vi "Dashboard Main.vi"() -> ()   [LabVIEW 2015]
uses:
  <vilib>/Utility/miscctls.llb/LVRowAndColumnTypeDef.ctl
  <vilib>/event_ctls.llb/eventvkey.ctl
  <vilib>/Rock Robotics/WPI/Dashboard/WPI_DashboardLogging Global.vi
  <vilib>/Rock Robotics/Network Tables/NT Read Numeric Array.vi
  <vilib>/Rock Robotics/Network Tables/NT Read Boolean.vi
  <vilib>/Utility/config.llb/Write Key (String).vi
  <vilib>/Utility/config.llb/Write Key (I32).vi
  <vilib>/Utility/config.llb/NI_LVConfig.lvlib
panel:
  in  "TCP":refnum<k5>
  in  "Rec Mode":enum32{"Stop", "Record", "Playback"}(radio)
  in  "Vision":u16(ring) items=["Camera Off", "USB Camera SW", "USB Camera HW", "IP Camera"]
  out "Camera IP":string
  out "Image Message":string="Timeout in Camera Communications"
  in  "Dashboard Tab":T1(tab)
  in  "Select Auto":string(combo)
  out "NT Connection":bool
  in  "Camera Settings":T2={"Frame Rate"=30, "Compression"=30, "Size"=1} {"Frame Rate" scale=1.0..30.0; "Size" items=["640x480", "320x240", "160x120"]}
  out "MotorChart R":cluster{"Numeric":dbl, "Numeric":dbl}(graph)
  out "MotorChart L":T3(graph)
  out "MotorSliders R":cluster{"MotorSlide1":dbl, "MotorSlide2":dbl} {"MotorSlide2" scale=-1.0..1.0 scale format="%#_2e"; "MotorSlide1" scale=-1.0..1.0 scale format="%#_2e"}
  out "MotorSliders L":T4 {"MotorSlide4 2" scale=0.0..14.0 scale format="%#_2e"; "MotorSlide2" scale=-1.0..1.0 scale format="%#_2e"; "MotorSlide1" scale=-1.0..1.0 scale format="%#_2e"}
  out "Gyro":dbl(knob) scale=0.0..360.0
  out "JS1 Z":dbl(slide) scale=-1.0..1.0 scale format="%#_2e"
  out "JS1 Graph":cluster{"X":dbl, "Y":dbl}[](graph)
  out "JS1 Buttons":T5
  out "JS2 Z":dbl(slide) scale=-1.0..1.0 scale format="%#_2e"
  out "JS2 Graph":cluster{"X":dbl, "Y":dbl}[](graph)
  out "JS2 Buttons":T5
  out "Mode":T6(ring)=enum."Auto Disabled"
  in  "DB Camera Config":bool
  out "fps":dbl format="%#.1g"
  out "Mbps":dbl format="%#.1g"
  out "Mbps LED":bool
  in  "DB/String 9":string
  in  "DB/String 8":string
  in  "DB/String 7":string
  in  "DB/String 6":string
  in  "DB/String 5":string
  in  "DB/String 4":string
  in  "DB/String 3":string
  in  "DB/String 2":string
  in  "DB/String 1":string
  in  "DB/String 0":string
  in  "DB/Slider 0":dbl(slide) scale=0.0..5.0
  in  "DB/Slider 1":dbl(slide) scale=0.0..5.0
  in  "DB/Slider 2":dbl(slide) scale=0.0..5.0
  in  "DB/Slider 3":dbl(slide) scale=0.0..5.0
  out "DB/LED 3":bool
  out "DB/LED 2":bool
  out "DB/LED 1":bool
  out "DB/LED 0":bool
  in  "DB/Button 3":bool
  in  "DB/Button 2":bool
  in  "DB/Button 1":bool
  in  "DB/Button 0":bool caption="New Name"
  out "Target In Range":bool
  out "Target Found":bool
  out "Auto Aim Running":bool
  out "Target Position":string
  out "Target Distance":dbl
  in  "Auto Select":i32(knob) scale=0.0..10.0
  out "Shooter Ready":bool
  out "Vision FPS":dbl
  out "Auto Aim Ready":bool
  in  "Test Slider":dbl(slide) scale=0.0..100.0 scale format="%#_3g"
  in  "On/Off":bool caption="Solenoid"
  in  "Test Name":u16(ring) items=["Select the test to run..."]
  in  "Test Tree":string(tree)
  in  "Motor":cluster{"Value":dbl, "Enable":bool} {"Value" scale=-1.0..1.0 scale format="%#_3g"}
  out "Progress":T7 {"Test Progress" scale=0.0..100.0}
  in  "Rev/Fwd":cluster{"Forward":bool, "Reverse":bool}
  in  "Test Ring":u16(ring) items=["Monochrome", "Color"]
  out "Cmd Status":string
  in  "Execute Command":bool
  in  "Command Params":string[][](table)
  in  "Command Selection":i32(listbox)
  in  "CheckList":i32(listbox)
  out "Tree":string(tree)
  out "Camera Image":T8(plugin-control)
  out "Background":bool
  # "Left"
  # "Front"
  # "Right"
  # "Battery"
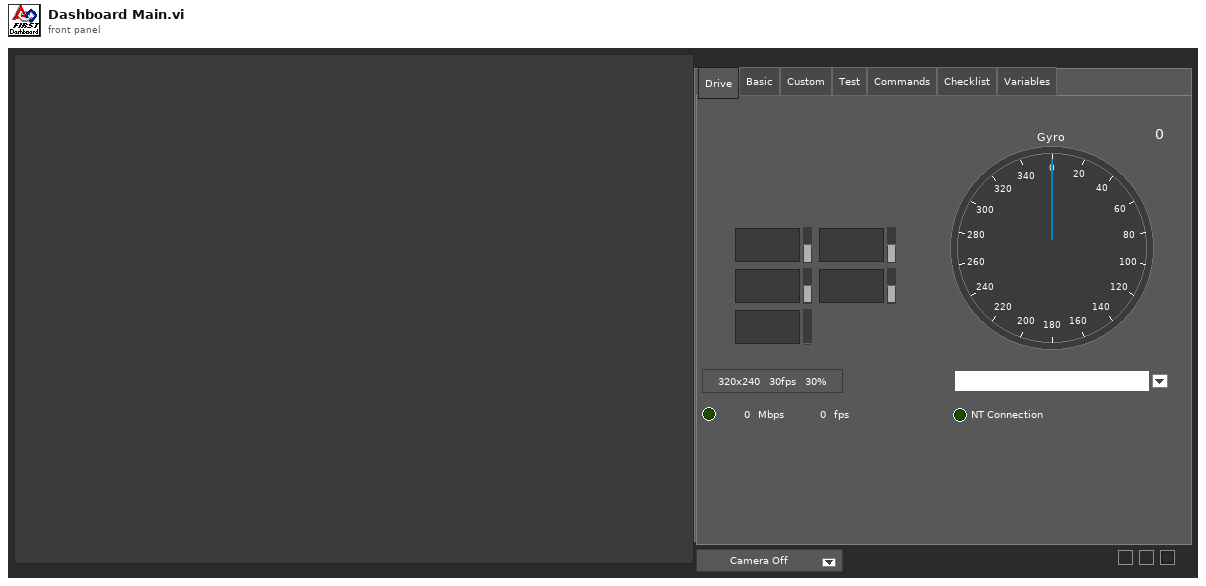
[diagram p1: front panel]
types:
  T1 = enum32{"Drive", "Basic", "Custom", "Test", "Commands", "Checklist", "Variables"}
  T2 = cluster{"Frame Rate":i32, "Compression":i32, "Size":u16}
  T3 = cluster{"Numeric":dbl, "Numeric":dbl, "Battery V":dbl}
  T4 = cluster{"MotorSlide1":dbl, "MotorSlide2":dbl, "MotorSlide4 2":dbl}
  T5 = cluster{bool, bool, bool, bool, bool, bool, bool, bool, bool, bool, bool, bool}
  T6 = enum8{"Tele-Op Disabled", "Tele-Op Enabled", "Auto Disabled", "Auto Enabled", "Test Disabled", "Test Enabled", "Disconnected", "No Code", "E-Stop"}
  T7 = cluster{"Test Progress":u8, "Test Progress Text":string}
  T8 = typedef "IMAQ Image.ctl" = refnum<image>
  T9 = cluster{"IDs":cluster{"RPC field ID":u16, "Unique ID":u16}, "String":string}
  T10 = enum32{"Drive", "Basic", "Custom", "Test", "Checklist", "Variables"}
  T11 = typedef "Image Type" = u32
  T12 = cluster{"Camera Image":refnum<vi>, "Dashboard Tab":refnum<vi>, "Background":refnum<vi>, "Vision":refnum<vi>, "Rec Mode":refnum<vi>, "Test Slider":refnum<vi>, "On/Off ":refnum<vi>, "Test Ring":refnum<vi>, "Rev/Fwd":refnum<vi>, "Test Name":refnum<vi>, "Motor":refnum<vi>, "Progress":refnum<vi>, "CheckList":refnum<vi>, "Tree":refnum<vi>, "Test Tree":refnum<vi>, "Command Params":refnum<vi>, "Command Selection":refnum<vi>, "Execute Command":refnum<vi>, "Cmd Status":refnum<vi>}
  T13 = cluster{"Error Strings":string, "Disable Counts":cluster{u16, u16}, "Rail Faults":cluster{u16, u16, u16}, "Robot IP":string, "DB Mode":u8, "Event Info":cluster{"Name":string, "Type":u8, "Number":u16, "Replay":u8}, "Camera Addr":string}
  T14 = cluster{"Storage":cluster{"Disk Free":u64, "RAM Block":u32, "RAM free":u32}, "CPU Utilization":cluster{"CPU % ISR":sgl, "CPU % Time Crit":sgl, "CPU % Timed Str":sgl, "CPU % High":sgl, "CPU % Above":sgl, "CPU % Normal":sgl, "CPU % Low":sgl}, "CAN":cluster{"% Bus Utilization":sgl, "Bus Off Cnt":u32, "TX_FIFO Full Cnt":u32, "Receive Error Cnt":u8, "Transmit Error Cnt":u8}, "HID":cluster{"HID Outputs":u32, "Rumble Low":u16, "Rumble High":u16}[]}
  T15 = cluster{"Status bits":cluster{"Test Mode":bool, "Autonomous":bool, "Enabled":bool, "Code Start":bool, "Brownout":bool, "Reserved 2":bool, "Reserved 3":bool, "E-Stop":bool}, "Code Trace":cluster{"Disabled":bool, "TeleOp":bool, "Auto":bool, "Test":bool}, "Controller Type":enum16{"unknown", "cRIO", "roboRio"}, "Code?":enum16{"unknown", "noCode", "code"}, "Battery V":dbl}
  T16 = cluster{"Control Bits":cluster{"TestMode":bool, "Autonomous":bool, "Enabled":bool, "FMS Present":bool, bool, bool, bool, "E-Stop":bool}, "Team Station ":u8, "Countdown":sgl, "Joystick Values":cluster{"Axes":dbl[], "Buttons":bool[], "POVs":i16[]}[]}
  T17 = cluster{"Axes":dbl[], "Buttons":bool[], "POVs":i16[]}[]
  T18 = cluster{"Axes":dbl[], "Buttons":bool[], "POVs":i16[]}
  T19 = cluster{"Buttons[0]":bool, "Buttons[1]":bool, "Buttons[2]":bool, "Buttons[3]":bool, "Buttons[4]":bool, "Buttons[5]":bool, "Buttons[6]":bool, "Buttons[7]":bool, "Buttons[8]":bool, "Buttons[9]":bool, "Buttons[10]":bool, "Buttons[11]":bool}
  T20 = typedef "NI_LVConfig.lvlib/Config Data RefNum.ctl" = refnum<k1>
  T21 = cluster{"Operation":enum16{"Update", "Clear"}, "Color Box":u32}[]
  T22 = typedef "eventvkey.ctl" = enum16{"ASCII", "Enter", "Return", "Shift", "Ctrl", "Alt", "Cmd", "Opt", "Caps", "NumLock", "Clear", "Break", "Up", "Down", "Left", "Right", "Insert", "Delete", "Home", "End", "PageUp", "PageDown", "Escape", "Help", "Pause", "ScrollLock", "F1", "F2", "F3", "F4", "F5", "F6", "F7", "F8", "F9", "F10", "F11", "F12", "F13", "F14", "F15", "F16", "F17", "F18", "F19", "F20", "F21", "F22", "F23", "F24", "Play", "VolumeUp", "VolumeDown", "Mute", "Two Byte Char"}
  T23 = cluster{"Image Size":bool, "Image Type":bool, "Pixel Value":bool, "ROI Information":bool, "Zoom Factor":bool}
  T24 = enum8{"Enabled", "Disabled", "Disabled and Grayed Out"}
  T25 = cluster{"Operation":enum16{"Update", "Clear"}, "Color Box":u32}
  T26 = typedef "LVRowAndColumnTypeDef.ctl" = cluster{"Row":i32, "Column":i32}
  T27 = cluster{"Shift":bool, "Ctrl":bool, "Alt":bool, "Cmd":bool, "Opt":bool}
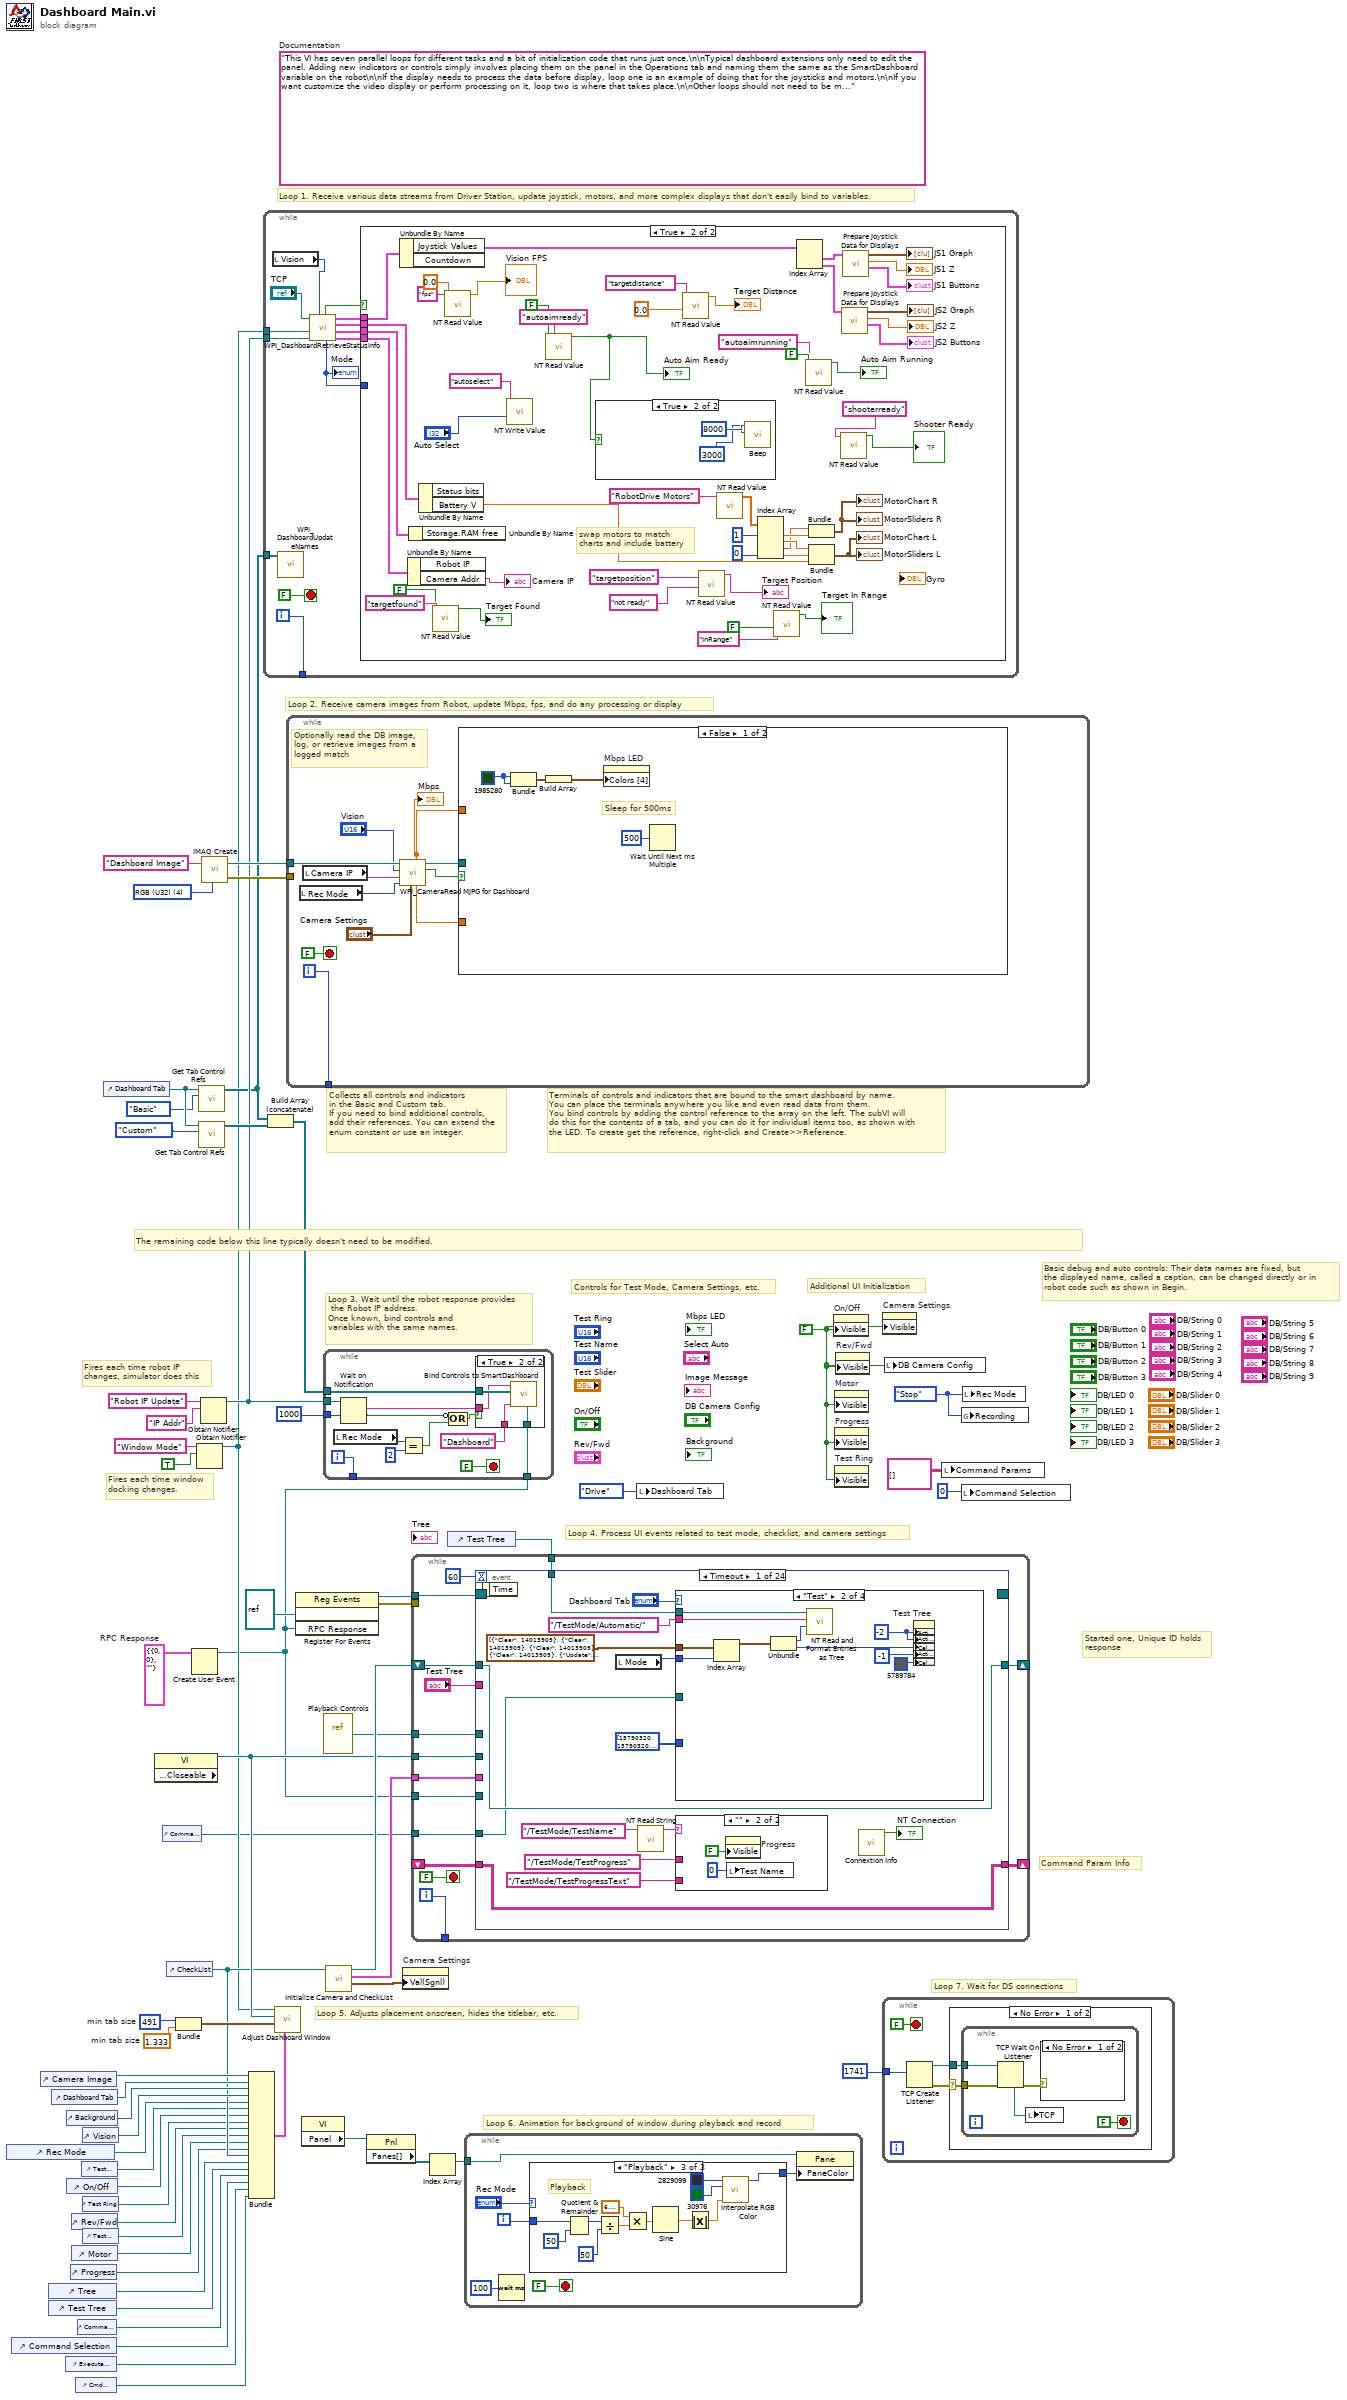
[diagram p0: block diagram]
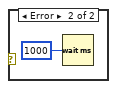
[diagram p2: hidden frame]
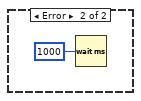
[diagram p3: hidden frame]
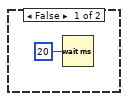
[diagram p4: hidden frame]
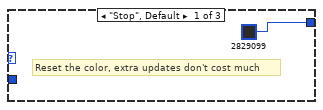
[diagram p6: hidden frame]
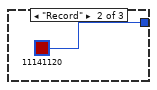
[diagram p7: hidden frame]
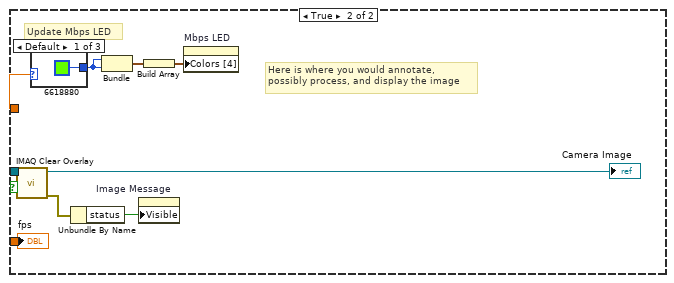
[diagram p9: hidden frame]
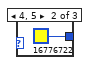
[diagram p10: hidden frame]
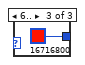
[diagram p11: hidden frame]
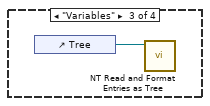
[diagram p13: hidden frame]
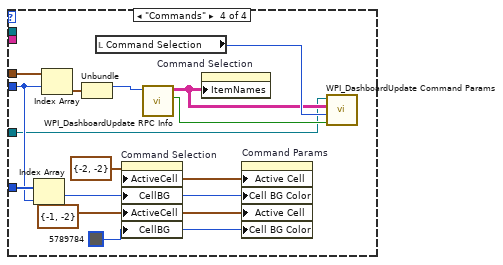
[diagram p14: hidden frame]
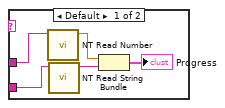
[diagram p15: hidden frame]
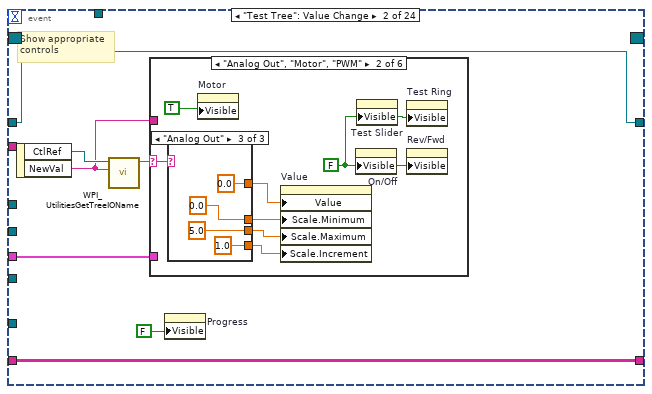
[diagram p16: hidden frame]
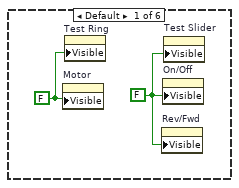
[diagram p17: hidden frame]
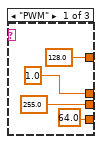
[diagram p18: hidden frame]
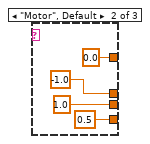
[diagram p19: hidden frame]
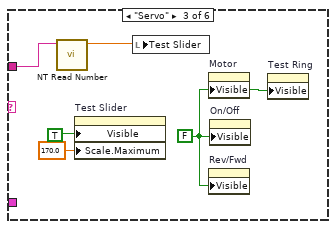
[diagram p20: hidden frame]
diagram:
  w7 = T9 {"IDs"={"RPC field ID"=0, "Unique ID"=0}, "String"=""}  # RPC Response
  w33 = 491  # min tab size
  w32 = 1.333  # min tab size
  w41 = enum32{"Stop", "Record", "Playback"}."Stop" ("Rec Mode")
  w15 = FALSE ("Visible")
  (unwired) "This VI has seven parallel loops for different tasks and a bit of initialization code that runs just once.\n\nTypical dashboard extensions only need to edit the panel. Adding new indicators or controls simply involves placing them on the panel in the Operations tab and naming them the same as the SmartDashboard variable on the robot\n\nIf the display needs to process the data before display, loop one is an example of doing that for the joysticks and motors.\n\nIf you want customize the video display or perform processing on it, loop two is where that takes place.\n\nOther loops should not need to be modified. They are pretty standard, and document the task they perform."  # Documentation
  w61 = T11 4 items=["Grayscale (U8)", "Grayscale (I16)", "Grayscale (SGL)", "Complex (CSG)", "RGB (U32)", "HSL (U32)", "RGB (U64)"] ("Image Type")
  # "Command Param Info"
  # "Started one, Unique ID holds\nresponse"
  # "Loop 7. Wait for DS connections"
  # "Basic debug and auto controls: Their data names are fixed, but\nthe displayed name, called a caption, can be changed directly or in\nrobot code such as shown in Begin."
  # "Controls for Test Mode, Camera Settings, etc."
  # "Additional UI Initialization"
  # "Loop 6. Animation for background of window during playback and record"
  # "Fires each time robot IP\nchanges, simulator does this"
  # "Fires each time window\ndocking changes."
  # "Collects all controls and indicators\nin the Basic and Custom tab.\nIf you need to bind additional controls,\nadd their references. You can extend the\nenum constant or use an integer."
  # "The remaining code below this line typically doesn't need to be modified."
  # "Loop 4. Process UI events related to test mode, checklist, and camera settings"
  # "Terminals of controls and indicators that are bound to the smart dashboard by name.\nYou can place the terminals anywhere you like and even read data from them.\nYou bind controls by adding the control reference to the array on the left. The subVI will\ndo this for the contents of a tab, and you can do it for individual items too, as shown with\nthe LED. To create get the reference, right-click and Create>>Reference."
  # "Loop 3. Wait until the robot response provides\n the Robot IP address.\nOnce known, bind controls and\nvariables with the same names."
  # "Loop 5. Adjusts placement onscreen, hides the titlebar, etc."
  # "Loop 1. Receive various data streams from Driver Station, update joystick, motors, and more complex displays that don't easily bind to variables."
  # "Loop 2. Receive camera images from Robot, update Mbps, fps, and do any processing or display"
  n1 = control-ref of="Rec Mode"() -> (w21:refnum<vi>)
  n2 = control-ref of="Command Selection"() -> (w6:refnum<vi>)
  n3 = control-ref of="Camera Image"() -> (w36:refnum<vi>)
  n4 = control-ref of="Tree"() -> (w25:refnum<vi>)
  n5 = control-ref of="Test Tree"() -> (w24:refnum<vi>)
  n6 = control-ref of="Dashboard Tab"() -> (w35:refnum<vi>)
  n7 = control-ref of="Execute Command"() -> (w8:refnum<vi>)
  n8 = control-ref of="Background"() -> (w30:refnum<vi>)
  n9 = control-ref of="On/Off"() -> (w19:refnum<vi>)
  n10 = control-ref of="Progress"() -> (w16:refnum<vi>)
  n11 = control-ref of="Rev/Fwd"() -> (w17:refnum<vi>)
  n12 = control-ref of="Motor"() -> (w22:refnum<vi>)
  n13 = control-ref of="Cmd Status"() -> (w2:refnum<vi>)
  n14 = control-ref of="Command Params"() -> (w9:refnum<vi>)
  n15 = control-ref of="Test Slider"() -> (w20:refnum<vi>)
  n16 = control-ref of="Vision"() -> (w34:refnum<vi>)
  n17 = control-ref of="Test Ring"() -> (w18:refnum<vi>)
  n18 = control-ref of="Test Name"() -> (w23:refnum<vi>)
  n19 = control-ref of="Dashboard Tab"() -> (w39:refnum<vi>)
  n20 = property class="VI" props=["Front Panel.Closeable"]() -> (reference out=w40:refnum<vi>)  [unwired: 2 in, 2 out]
  n21 = control-ref of="Command Params"() -> (w1:refnum<vi>)
  n22 = control-ref of="CheckList"() -> (w26:refnum<vi>)
  n23 = Bundle("min tab size"=w33, "min tab size"=w32) -> (w31:cluster{"min tab size":i32, "min tab size":dbl})  [unwired: 1 in]
  n24 = Create User Event(user event datatype=w7) -> (user event=w3:refnum<user-event>)  [unwired: 1 in, 1 out]
  n25 = Obtain Notifier(name (unnamed)="Window Mode", notification data type=TRUE) -> (notifier out=w12:refnum<notifier>)  [unwired: 2 in, 2 out]
  n26 = call <vilib>:"Get Tab Control Refs.vi"("Page Index"=T10."Basic" ("Dashboard Tab"), "TabControl in"=w39) -> ("ControlsOnPage"=w13:refnum<vi>[])  [unwired: 9 in]
  n27 = call <vilib>:"Get Tab Control Refs.vi"("Page Index"=T10."Custom" ("Dashboard Tab"), "TabControl in"=w39) -> ("ControlsOnPage"=w38:refnum<vi>[])  [unwired: 9 in]
  n28 = Obtain Notifier(name (unnamed)="Robot IP Update", notification data type="IP Addr" ("name (unnamed)")) -> (notifier out=w14:refnum<notifier>)  [unwired: 2 in, 2 out]
  n29 = call "IMAQ Create"("Image Name"="Dashboard Image", "Image Type"=w61) -> ("New Image"=w59:T8, "error out"=w58:errorcluster)  [unwired: 2 in, 1 out]
  n30 = Bundle("Camera Image"=w36, "Dashboard Tab"=w35, "Background"=w30, "Vision"=w34, "Rec Mode"=w21, "Test Slider"=w20, "On/Off"=w19, "Test Ring"=w18, "Rev/Fwd"=w17, "Test Name"=w23, "Motor"=w22, "Progress"=w16, "CheckList"=w26, "Tree"=w25, "Test Tree"=w24, "Command Params"=w9, "Command Selection"=w6, "Execute Command"=w8, "Cmd Status"=w2) -> (w27:T12)  [unwired: 1 in]
  n31 = while {
    tunnel: [w73] -> _
    tunnel: w14 -> [w67]
    tunnel: w13 -> [w66]
    tunnel: w12 -> [w62]
    i -> [w73]
    stop <- FALSE stop-if-true
    n32 = local read "Vision"() -> (w64:u16)
    n33 = call <vilib>:"WPI_DashboardUpdateNames.vi"("Controls on Tab"=w66) -> ()  [unwired: 11 in]
    n34 = call <vilib>:"WPI_DashboardRetrieveStatusInfo.vi"("Vision"=w64, "Binding Refnum"=w67, "Window Mode Notifier"=w62, "TCP Cnx"="TCP") -> ("Power and Errors"=w68:T13, "Robot Metrics"=w71:T14, "Status Info"=w72:T15, "Control Info"=w69:T16, "Robot Mode"=w65:T6, "Process?"=w70:bool)  [unwired: 2 in]
    "Mode" <- w65
    n35 = case shown="True" w70 {
      tunnel: w72 -> [_ w125]
      tunnel: w71 -> [_ w124]
      tunnel: w69 -> [_ w123]
      tunnel: w68 -> [_ w122]
      tunnel: w65 -> [_ _]
      frame False {
        n36 = Wait (ms)(milliseconds to wait=u32 20) -> ()  [unwired: 1 out]
      }
      frame True {
        # "swap motors to match\ncharts and include battery"
        n37 = Unbundle By Name(w123) -> ("Joystick Values"=w112:T17)  [unwired: 1 out]
        n38 = Unbundle By Name(w122) -> ("Camera Addr"=→"Camera IP":string)  [unwired: 1 out]
        n39 = Unbundle By Name(w124) -> ()  [unwired: 1 out]
        n40 = Unbundle By Name(w125) -> ("Battery V"=w113:dbl)  [unwired: 1 out]
        n41 = call-poly <vilib>:"NT Read Value.vi"("Default Value"=FALSE, "Name"="targetfound") -> ("Boolean"=→"Target Found":bool)  [unwired: 8 in, 1 out]
        n42 = call-poly <vilib>:"NT Read Value.vi"("Default Value"=0.0, "Name"="fps") -> ("Numeric"=→"Vision FPS":dbl)  [unwired: 8 in, 1 out]
        n43 = call-poly <vilib>:"NT Write Value.vi"("Numeric"="Auto Select", "Name"="autoselect") -> ()  [unwired: 9 in, 1 out]
        n44 = call-poly <vilib>:"NT Read Value.vi"("Default Value"=FALSE, "Name"="autoaimready") -> ("Boolean"=w97:bool)  [unwired: 8 in, 1 out]
        "Auto Aim Ready" <- w97
        n45 = case shown="True" w97 {
          frame False {
          }
          frame True {
            n46 = call <vilib>:"Beep.vi"("duration (msec)"=3000, "frequency (Hz)"=8000) -> ()  [unwired: 10 in]
          }
        }
        n47 = call-poly <vilib>:"NT Read Value.vi"("Default Value"=0.0, "Name"="targetdistance") -> ("Numeric"=→"Target Distance":dbl)  [unwired: 8 in, 1 out]
        n48 = call-poly <vilib>:"NT Read Value.vi"("Default Value"="not ready", "Name"="targetposition") -> ("String"=→"Target Position":string)  [unwired: 8 in, 1 out]
        n49 = call-poly <vilib>:"NT Read Value.vi"("Name"="RobotDrive Motors") -> ("Numeric Array"=w101:dbl[])  [unwired: 9 in, 1 out]
        n50 = Index Array(array=w101, index #1=1, index #4=0) -> (element #1=w117:dbl, element #2=w118:dbl, element #3=w116:dbl, element #4=w121:dbl)  [unwired: 2 in]
        n51 = call-poly <vilib>:"NT Read Value.vi"("Default Value"=FALSE, "Name"="InRange") -> ("Boolean"=→"Target In Range":bool)  [unwired: 8 in, 1 out]
        n52 = Index Array(array=w112) -> (element #1=w111:T18, element #2=w106:T18)  [unwired: 2 in]
        n53 = call-poly <vilib>:"NT Read Value.vi"("Default Value"=FALSE, "Name"="autoaimrunning") -> ("Boolean"=→"Auto Aim Running":bool)  [unwired: 8 in, 1 out]
        n54 = Bundle("Numeric"=w116, "Numeric"=w117) -> (→"MotorChart R" →"MotorSliders R":cluster{"Numeric":dbl, "Numeric":dbl})  [unwired: 1 in]
        n55 = Bundle("Numeric"=w118, "Numeric"=w121, "Battery V"=w113) -> (→"MotorChart L" →"MotorSliders L":T3)  [unwired: 1 in]
        n56 = call-poly <vilib>:"NT Read Value.vi"("Name"="shooterready") -> ("Boolean"=→"Shooter Ready":bool)  [unwired: 9 in, 1 out]
        n57 = call "Prepare Joystick Data for Displays.vi"("Joystick Values"=w106) -> ("Buttons"=→"JS2 Buttons":T19, "Z Axis"=→"JS2 Z":dbl, "Cartesian Data"=→"JS2 Graph":cluster{"X axis":dbl, "X axis":dbl}[])  [unwired: 8 in]
        n58 = call "Prepare Joystick Data for Displays.vi"("Joystick Values"=w111) -> ("Buttons"=→"JS1 Buttons":T19, "Z Axis"=→"JS1 Z":dbl, "Cartesian Data"=→"JS1 Graph":cluster{"X axis":dbl, "X axis":dbl}[])  [unwired: 8 in]
      }
    }
  }
  n59 = Build Array (concatenate)(w13, w38) -> (w37:refnum<vi>[])
  n60 = call "Adjust Dashboard Window.vi"("Sizing Refnums"=w27, "Size Constraints"=w31, "VI"=w40, "WIn Mode"=w12) -> ()  [unwired: 8 in]
  n61 = while {
    tunnel: w59 -> [w136]
    tunnel: w58 -> [_]
    tunnel: [w137] -> _
    i -> [w137]
    stop <- FALSE stop-if-true
    # "Optionally read the DB image,\nlog, or retrieve images from a\nlogged match"
    n62 = local read "Rec Mode"() -> (w131:enum32{"Stop", "Record", "Playback"})
    n63 = local read "Camera IP"() -> (w129:string)
    n64 = call <vilib>:"WPI_CameraRead MJPG for Dashboard.vi"("Camera Settings"="Camera Settings", "Rec Mode"=w131, "Camera IP"=w129, "Camera Mode"="Vision", "Refnum in"=w136) -> ("Active"=w134:bool, "Refnum out"=w135:T8, "FPS"=w133:dbl, "Bandwidth (Mbps)"=w128:dbl)  [unwired: 3 in]
    "Mbps" <- w128
    n65 = case shown="False" w134 {
      tunnel: w135 -> [_ w146]
      tunnel: w128 -> [_ w145]
      tunnel: w133 -> [_ w143]
      frame False {
        w139 = u32 1985280 ("Color Box")
        # "Sleep for 500ms"
        n66 = Bundle("Color Box"=w139, "Color Box"=w139) -> (w141:cluster{"Color Box":u32, "Color Box":u32})  [unwired: 1 out]
        n67 = Build Array(w141) -> (w140:cluster{"Color Box":u32, "Color Box":u32}[])
        n68 = property on="Mbps LED" class="Bool (strict)"("Colors [4]"=w140) -> ()  [unwired: 2 in, 2 out]
        n69 = Wait Until Next ms Multiple(millisecond multiple=u32 500) -> ()  [unwired: 1 out]
      }
      frame True {
        # "Here is where you would annotate,\npossibly process, and display the image"
        # "Update Mbps LED"
        n70 = call "IMAQ Clear Overlay"("Image"=w146) -> ("error out"=w150:errorcluster, "Image Out"=→"Camera Image":T8)  [unwired: 2 in, 7 out]
        n71 = case shown="Default" w145 {
          tunnel: [u32 6618880 ("Color Box") u32 16776722 ("Color Box") u32 16716800 ("Color Box")] -> w147
          frame Default {
          }
          frame 4, 5 {
          }
          frame 6.. {
          }
        }
        n72 = Unbundle By Name(w150) -> ("status"=w151:bool)
        n73 = Bundle("Color Box"=w147, "Color Box"=w147) -> (w149:cluster{"Color Box":u32, "Color Box":u32})  [unwired: 1 out]
        n74 = property on="Image Message" class="Str"("Visible"=w151) -> ()  [unwired: 2 in, 2 out]
        n75 = Build Array(w149) -> (w148:cluster{"Color Box":u32, "Color Box":u32}[])
        n76 = property on="Mbps LED" class="Bool (strict)"("Colors [4]"=w148) -> ()  [unwired: 2 in, 2 out]
        "fps" <- w143
      }
    }
  }
  n77 = register-events(refnum<vi> refnum, w3) -> (reference out=w45:refnum<event-registration>, error out=w44:errorcluster)  [unwired: 2 in]
  n78 = property class="VI"() -> ("Panel"=w48:refnum<vi>)  [unwired: 2 in, 2 out]
  n79 = while {
    tunnel: w37 -> [w167]
    tunnel: w14 -> [w165]
    tunnel: [w163] -> _
    tunnel: u32 1000 ("milliseconds to wait") -> [w162]
    tunnel: w3 -> [w155]
    i -> [w163]
    stop <- FALSE stop-if-true
    n80 = local read "Rec Mode"() -> (w158:enum32{"Stop", "Record", "Playback"})
    n81 = Wait on Notification(notifier=w165, timeout in ms (-1)=w162) -> (notification=w164:string, timed out?=w160:bool)  [unwired: 2 in, 2 out]
    n82 = Equal?(x=w158, y=u16 2 ("Rec Mode")) -> (x = y?=w159:bool)
    n83 = Compound Arithmetic op=OR(invert w160, w159) -> (w161:bool)
    n84 = case shown="True" w161 {
      tunnel: w167 -> [_ w171]
      tunnel: w164 -> [_ w170]
      tunnel: "Dashboard" -> [_ w169]
      tunnel: w155 -> [_ w168]
      frame False {
      }
      frame True {
        n85 = call <vilib>:"Bind Controls to SmartDashboard.vi"("RPC ref"=w168, "Client Name"=w169, "Bound Control Refs"=w171, "Server IP Address"=w170) -> ()  [unwired: 8 in]
      }
    }
  }
  n86 = vi-ref "Playback Controls.vi"() -> (w46:refnum<vi>)
  n87 = call "Initialize Camera and CheckList.vi"("ListBox in"=w26) -> ("Cluster"=w52:cluster{"value":i32, "value":i32, "index":i32}, "Array"=w53:cluster{string[]}[], "File Refnum"=w51:T20)  [unwired: 8 in]
  n88 = property class="Pnl"(reference=w48) -> ("Panes[]"=w49:refnum<vi>[])  [unwired: 1 in, 2 out]
  n89 = property on="Camera Settings" class="Clust (strict)"("Val(Sgnl)"=w52) -> ()  [unwired: 2 in, 2 out]
  n90 = Index Array(array=w49) -> (element=w47:refnum<vi>)  [unwired: 1 in]
  n91 = control-ref of="Test Tree"() -> (w50:refnum<vi>)
  n92 = while {
    tunnel: w53 -> [w183]
    shift-right: [w182] -> _
    shift-left: w51 -> [w181]
    tunnel: [w180] -> _
    tunnel: w50 -> [w179]
    tunnel: w46 -> [w178]
    tunnel: w45 -> [w177]
    tunnel: w44 -> [_]
    tunnel: w40 -> [w176]
    tunnel: w3 -> [w175]
    tunnel: w1 -> [w174]
    shift-right: [w173] -> _
    shift-left: _ -> [w172]
    i -> [w180]
    stop <- FALSE stop-if-true
    n93 = event shown="[0] Timeout" {
      selector: w177 -> [_ _ _ _ _ _ _ _ _ _ _ _ _ _ _ _ _ _ _ _ _ _ _ _]
      dyn-events: [_ _ _ _ _ _ _ _ _ _ _ _ _ _ _ _ _ _ w492 _ _ _ _ _] -> _
      timeout: u32 60 ("milliseconds to wait") -> [_ _ _ _ _ _ _ _ _ _ _ _ _ _ _ _ _ _ _ _ _ _ _ _]
      tunnel: w179 -> [w196 _ _ _ _ _ _ _ _ _ _ _ _ _ _ _ _ _ _ _ _ _ _ _]
      tunnel: "Test Tree" -> [_ _ _ _ _ _ _ _ _ _ _ _ _ w455 w464 w467 w472 w481 _ _ _ _ _ _]
      tunnel: w183 -> [_ w234 _ _ _ _ _ _ _ _ _ w417 w448 _ _ _ _ _ _ _ _ _ _ _]
      tunnel: [w193 w233 w337 w343 w353 w357 w363 w375 w383 w389 w402 w416 w441 w454 w462 w466 w471 w480 w494 w510 w512 w520 w531 w536] -> w182
      tunnel: w181 -> [w193 w233 w337 w343 w353 w357 w363 w375 w383 w389 w402 w415 w441 w454 w462 w466 w471 w480 w494 w510 w512 w520 w531 w536]
      tunnel: w178 -> [_ _ _ _ _ _ _ _ _ _ _ _ _ _ _ _ _ _ w495 _ w515 _ _ _]
      tunnel: w176 -> [_ _ _ _ _ _ _ _ _ _ _ _ _ _ _ _ _ _ w490 _ _ _ _ _]
      tunnel: w175 -> [_ _ _ _ _ _ _ _ _ _ _ _ _ _ _ _ _ _ w486 _ _ _ _ _]
      tunnel: w174 -> [w188 _ _ _ _ _ w361 _ _ _ _ _ _ _ _ _ _ _ _ _ _ _ _ _]
      tunnel: [w187 w232 w336 w342 w352 w358 w359 w369 w380 w388 w401 w414 w440 w453 w461 w465 w470 w479 w485 w508 w511 w516 w524 w537] -> w173
      tunnel: w172 -> [w187 w232 w336 w342 w352 w358 w359 _ _ w388 w401 w414 w440 w453 w461 w465 w470 w479 w485 w508 w511 w516 w524 w537]
      event Timeout {
        n94 = event-data() -> ()  [unwired: 1 in, 1 out]
        n95 = local read "Mode"() -> (w190:T6)
        n96 = call <vilib>:"NT Read String.vi"("Name"="/TestMode/TestName") -> ("String"=w199:string)  [unwired: 9 in, 1 out]
        n97 = case shown="\"Test\"" "Dashboard Tab" {
          tunnel: w196 -> [_ w210 _ _]
          tunnel: "/TestMode/Automatic/" ("Name Pattern") -> [_ w209 _ _]
          tunnel: T21 [{"Operation"=enum."Clear", "Color Box"=14013909}, {"Operation"=enum."Clear", "Color Box"=14013909}, {"Operation"=enum."Clear", "Color Box"=14013909}, {"Operation"=enum."Clear", "Color Box"=14013909}, {"Operation"=enum."Update", "Color Box"=14013909}, {"Operation"=enum."Update", "Color Box"=16777215}, {"Operation"=enum."Clear", "Color Box"=14013909}, {"Operation"=enum."Clear", "Color Box"=14013909}, {"Operation"=enum."Clear", "Color Box"=14013909}] -> [_ w202 _ w219]
          tunnel: w190 -> [_ w201 _ w218]
          tunnel: u32[] [15790320, 15790320, 15790320, 15790320, 16777215, 16777215, 15790320, 15790320, 15790320] -> [_ _ _ w224]
          tunnel: w188 -> [_ _ _ w212]
          frame "Custom", Default {
          }
          frame "Test" {
            w208 = -2 ("Active Item:Row Number")
            n98 = Index Array(array=w202, index=w201) -> (element=w203:T25)
            n99 = Unbundle(w203) -> ("Operation"=w204:enum16{"Update", "Clear"}, "Color Box"=w205:u32)
            n100 = call <vilib>:"NT Read and Format Entries as Tree.vi"("Operation"=w204, "Name Pattern"=w209, "Tree Refnum"=w210) -> ()  [unwired: 7 in, 2 out]
            n101 = property on="Test Tree" class="Tree (strict)"("Active Item Row Number"=w208, "ActiveColNum"=w208, "CellBG"=w205, "Active Item Row Number"=-1 ("Active Item:Row Number"), "CellBG"=u32 5789784 ("Color Box")) -> ()  [unwired: 2 in, 2 out]
          }
          frame "Variables" {
            n102 = control-ref of="Tree"() -> (w211:refnum<vi>)
            n103 = call <vilib>:"NT Read and Format Entries as Tree.vi"("Tree Refnum"=w211) -> ()  [unwired: 9 in, 2 out]
          }
          frame "Commands" {
            w220 = u32 5789784 ("Color Box")
            w221 = T26 {"Row"=-1, "Column"=-2} ("Active Cell:Active Cell")
            w223 = T26 {"Row"=-2, "Column"=-2} ("Active Cell:Active Cell")
            n104 = Index Array(array=w224, index=w218) -> (element=w222:u32)
            n105 = Index Array(array=w219, index=w218) -> (element=w217:T25)
            n106 = Unbundle(w217) -> ("Operation"=w216:enum16{"Update", "Clear"})  [unwired: 1 out]
            n107 = local read "Command Selection"() -> (w215:i32)
            n108 = property on="Command Selection" class="MCListbox (strict)"("ActiveCell"=w223, "CellBG"=w222, "ActiveCell"=w221, "CellBG"=w220) -> ()  [unwired: 2 in, 2 out]
            n109 = call <vilib>:"WPI_DashboardUpdate RPC Info.vi"("Operation"=w216) -> ("update"=w214:bool, "commands"=w213:string[][])  [unwired: 9 in]
            n110 = property on="Command Selection" class="MCListbox (strict)"("ItemNames"=w213) -> ()  [unwired: 2 in, 2 out]
            n111 = property on="Command Params" class="Tbl (strict)"("Active Cell"=w223, "Cell BG Color"=w222, "Active Cell"=w221, "Cell BG Color"=w220) -> ()  [unwired: 2 in, 2 out]
            n112 = call <vilib>:"WPI_DashboardUpdate Command Params.vi"("Update"=w214, "NewVal"=w215, "Commands"=w213, "Param Tbl"=w212) -> ()  [unwired: 7 in, 1 out]
          }
        }
        n113 = case shown="\"\"" w199 {
          tunnel: "/TestMode/TestProgress" ("Name") -> [w226 _]
          tunnel: "/TestMode/TestProgressText" ("Name") -> [w225 _]
          frame Default {
            n114 = call <vilib>:"NT Read Number.vi"("Name"=w226) -> ("Numeric"=w227:dbl)  [unwired: 9 in, 1 out]
            n115 = call <vilib>:"NT Read String.vi"("Name"=w225) -> ("String"=w228:string)  [unwired: 9 in, 1 out]
            n116 = Bundle("Numeric"=w227, "String"=w228) -> (→"Progress":cluster{"Numeric":dbl, "String":string})  [unwired: 1 in]
          }
          frame "" {
            n117 = property on="Progress" class="Clust (strict)"("Visible"=FALSE) -> ()  [unwired: 2 in, 2 out]
            n118 = local write "Test Name"(u16 0) -> ()
          }
        }
        n119 = call <vilib>:"Connextion Info.vi"() -> ("Connected"=→"NT Connection":bool)  [unwired: 10 in, 1 out]
      }
      event "Test Tree": Value Change {
        # "Show appropriate\ncontrols"
        n120 = event-data() -> ("CtlRef"=w237:refnum<vi>, "NewVal"=w235:string)  [unwired: 1 in]
        n121 = call <vilib>:"WPI_UtilitiesGetTreeIOName.vi"("NewVal"=w235, "TreeControl in"=w237) -> ("I/O Name"=w238:string)  [unwired: 9 in]
        n122 = case shown="\"Analog Out\", \"Motor\", \"PWM\"" w238 {
          selector: w238 -> [_ w245 _ w267 w276 _]
          tunnel: w235 -> [_ _ w264 w266 _ w283]
          tunnel: w234 -> [_ _ _ _ _ w282]
          frame Default {
            w240 = FALSE ("Visible")
            w239 = FALSE ("Visible")
            n123 = property on="Motor" class="Clust (strict)"("Visible"=w239) -> ()  [unwired: 2 in, 2 out]
            n124 = property on="Test Ring" class="Ring (strict)"("Visible"=w239) -> ()  [unwired: 2 in, 2 out]
            n125 = property on="Rev/Fwd" class="Clust (strict)"("Visible"=w240) -> ()  [unwired: 2 in, 2 out]
            n126 = property on="On/Off" class="Bool (strict)"("Visible"=w240) -> ()  [unwired: 2 in, 2 out]
            n127 = property on="Test Slider" class="Slide (strict)"("Visible"=w240) -> ()  [unwired: 2 in, 2 out]
          }
          frame "Analog Out", "Motor", "PWM" {
            w246 = FALSE ("Visible")
            n128 = case shown="\"Analog Out\"" w245 {
              tunnel: [1.0 ("Value") -1.0 ("Value") 0.0 ("Value")] -> w244
              tunnel: [255.0 ("Value") 1.0 ("Value") 5.0 ("Value")] -> w243
              tunnel: [128.0 ("Value") 0.0 ("Value") 0.0 ("Value")] -> w242
              tunnel: [64.0 ("Value") 0.5 ("Value") 1.0 ("Value")] -> w241
              frame "PWM" {
              }
              frame "Motor", Default {
              }
              frame "Analog Out" {
              }
            }
            n129 = property on="Motor" class="Clust (strict)"("Visible"=TRUE) -> ()  [unwired: 2 in, 2 out]
            n130 = property on="Value" class="Slide (strict)"("Value"=w242, "Scale.Minimum"=w244, "Scale.Maximum"=w243, "Scale.Increment"=w241) -> ()  [unwired: 2 in, 2 out]
            n131 = property on="On/Off" class="Bool (strict)"("Visible"=w246) -> ()  [unwired: 2 in, 2 out]
            n132 = property on="Test Slider" class="Slide (strict)"("Visible"=w246) -> ()  [unwired: 2 in, 2 out]
            n133 = property on="Test Ring" class="Ring (strict)"("Visible"=w246) -> ()  [unwired: 2 in, 2 out]
            n134 = property on="Rev/Fwd" class="Clust (strict)"("Visible"=w246) -> ()  [unwired: 2 in, 2 out]
          }
          frame "Servo" {
            w262 = FALSE ("Visible")
            n135 = call <vilib>:"NT Read Number.vi"("Name"=w264) -> ("Numeric"=w263:dbl)  [unwired: 9 in, 1 out]
            n136 = property on="Test Slider" class="Slide (strict)"("Visible"=TRUE, "Scale.Maximum"=170.0 ("Scale.Range:Maximum")) -> ()  [unwired: 2 in, 2 out]
            n137 = local write "Test Slider"(w263) -> ()
            n138 = property on="Motor" class="Clust (strict)"("Visible"=w262) -> ()  [unwired: 2 in, 2 out]
            n139 = property on="Rev/Fwd" class="Clust (strict)"("Visible"=w262) -> ()  [unwired: 2 in, 2 out]
            n140 = property on="On/Off" class="Bool (strict)"("Visible"=w262) -> ()  [unwired: 2 in, 2 out]
            n141 = property on="Test Ring" class="Ring (strict)"("Visible"=w262) -> ()  [unwired: 2 in, 2 out]
          }
          frame "Relay", "Solenoid" {
            w265 = FALSE ("Visible")
            n142 = property on="Motor" class="Clust (strict)"("Visible"=w265) -> ()  [unwired: 2 in, 2 out]
            n143 = property on="Test Slider" class="Slide (strict)"("Visible"=w265) -> ()  [unwired: 2 in, 2 out]
            n144 = Search and Replace String(input string=w266, search string="/Value  **", replace string="/Direction") -> (result string=w272:string)  [unwired: 5 in, 3 out]
            n145 = property on="Test Ring" class="Ring (strict)"("Visible"=w265) -> ()  [unwired: 2 in, 2 out]
            n146 = call <vilib>:"NT Read String.vi"("Name"=w272) -> ("String"=w270:string)  [unwired: 9 in, 1 out]
            n147 = Equal?(x="Both directions", y=w270) -> (x = y?=w268:bool)
            n148 = Not(x=w268) -> (.not. x?=w269:bool)
            n149 = property on="Rev/Fwd" class="Clust (strict)"("Visible"=w268) -> ()  [unwired: 2 in, 2 out]
            n150 = property on="On/Off" class="Bool (strict)"("Visible"=w269, "Caption.Text"=w267) -> ()  [unwired: 2 in, 2 out]
          }
          frame "Compressor", "Digital Out" {
            w275 = FALSE ("Visible")
            # "Get direction and finish"
            n151 = property on="Motor" class="Clust (strict)"("Visible"=w275) -> ()  [unwired: 2 in, 2 out]
            n152 = property on="Test Slider" class="Slide (strict)"("Visible"=w275) -> ()  [unwired: 2 in, 2 out]
            n153 = property on="Test Ring" class="Ring (strict)"("Visible"=w275) -> ()  [unwired: 2 in, 2 out]
            n154 = property on="On/Off" class="Bool (strict)"("Visible"=TRUE, "Caption.Text"=w276) -> ()  [unwired: 2 in, 2 out]
            n155 = property on="Rev/Fwd" class="Clust (strict)"("Visible"=FALSE) -> ()  [unwired: 2 in, 2 out]
          }
          frame "Camera" {
            n156 = call <vilib>:"Get Last Path Segment.vi"("String in"=w283) -> ("String out"=w284:string)  [unwired: 10 in]
            n157 = property on="On/Off" class="Bool (strict)"("Visible"=FALSE) -> ()  [unwired: 2 in, 2 out]
            n158 = property on="Motor" class="Clust (strict)"("Visible"=FALSE) -> ()  [unwired: 2 in, 2 out]
            n159 = property on="Rev/Fwd" class="Clust (strict)"("Visible"=FALSE) -> ()  [unwired: 2 in, 2 out]
            n160 = case shown="\"White Balance  **\"" w284 {
              tunnel: w283 -> [w290 w299 w308 w317 w326 _ w332]
              tunnel: w282 -> [w288 w296 w305 w314 w323 _ _]
              frame "Size  **" {
                n161 = Index Array(array=w288) -> (element=w287:cluster{string[]})  [unwired: 1 in]
                n162 = call <vilib>:"NT Read String.vi"("Name"=w290) -> ("String"=w289:string)  [unwired: 9 in, 1 out]
                n163 = Unbundle(w287) -> (w285:string[])
                n164 = Match First String(2:w285, 3:w289) -> (0:w286:i32)  [unwired: 1 out]
                n165 = property on="Test Ring" class="Ring (strict)"("Value"=w286, "Strings []"=w285) -> ()  [unwired: 2 in, 2 out]
                n166 = property on="Test Ring" class="Ring (strict)"("Visible"=TRUE) -> ()  [unwired: 2 in, 2 out]
                n167 = property on="Test Slider" class="Slide (strict)"("Visible"=FALSE) -> ()  [unwired: 2 in, 2 out]
              }
              frame "White Balance  **" {
                n168 = Index Array(array=w296, index=1) -> (element=w297:cluster{string[]})
                n169 = call <vilib>:"NT Read String.vi"("Name"=w299) -> ("String"=w298:string)  [unwired: 9 in, 1 out]
                n170 = Unbundle(w297) -> (w294:string[])
                n171 = Match First String(2:w294, 3:w298) -> (0:w293:i32)  [unwired: 1 out]
                n172 = property on="Test Ring" class="Ring (strict)"("Value"=w293, "Strings []"=w294) -> ()  [unwired: 2 in, 2 out]
                n173 = property on="Test Ring" class="Ring (strict)"("Visible"=TRUE) -> ()  [unwired: 2 in, 2 out]
                n174 = property on="Test Slider" class="Slide (strict)"("Visible"=FALSE) -> ()  [unwired: 2 in, 2 out]
              }
              frame "Exposure  **" {
                n175 = Index Array(array=w305, index=2) -> (element=w306:cluster{string[]})
                n176 = call <vilib>:"NT Read String.vi"("Name"=w308) -> ("String"=w307:string)  [unwired: 9 in, 1 out]
                n177 = Unbundle(w306) -> (w302:string[])
                n178 = Match First String(2:w302, 3:w307) -> (0:w303:i32)  [unwired: 1 out]
                n179 = property on="Test Ring" class="Ring (strict)"("Value"=w303, "Strings []"=w302) -> ()  [unwired: 2 in, 2 out]
                n180 = property on="Test Ring" class="Ring (strict)"("Visible"=TRUE) -> ()  [unwired: 2 in, 2 out]
                n181 = property on="Test Slider" class="Slide (strict)"("Visible"=FALSE) -> ()  [unwired: 2 in, 2 out]
              }
              frame "Exposure Priority  **" {
                n182 = Index Array(array=w314, index=3) -> (element=w315:cluster{string[]})
                n183 = call <vilib>:"NT Read String.vi"("Name"=w317) -> ("String"=w316:string)  [unwired: 9 in, 1 out]
                n184 = Unbundle(w315) -> (w311:string[])
                n185 = Match First String(2:w311, 3:w316) -> (0:w312:i32)  [unwired: 1 out]
                n186 = property on="Test Ring" class="Ring (strict)"("Value"=w312, "Strings []"=w311) -> ()  [unwired: 2 in, 2 out]
                n187 = property on="Test Ring" class="Ring (strict)"("Visible"=TRUE) -> ()  [unwired: 2 in, 2 out]
                n188 = property on="Test Slider" class="Slide (strict)"("Visible"=FALSE) -> ()  [unwired: 2 in, 2 out]
              }
              frame "Color Enable  **" {
                n189 = Index Array(array=w323, index=4) -> (element=w324:cluster{string[]})
                n190 = call <vilib>:"NT Read String.vi"("Name"=w326) -> ("String"=w325:string)  [unwired: 9 in, 1 out]
                n191 = Unbundle(w324) -> (w320:string[])
                n192 = Match First String(2:w320, 3:w325) -> (0:w321:i32)  [unwired: 1 out]
                n193 = property on="Test Ring" class="Ring (strict)"("Value"=w321, "Strings []"=w320) -> ()  [unwired: 2 in, 2 out]
                n194 = property on="Test Ring" class="Ring (strict)"("Visible"=TRUE) -> ()  [unwired: 2 in, 2 out]
                n195 = property on="Test Slider" class="Slide (strict)"("Visible"=FALSE) -> ()  [unwired: 2 in, 2 out]
              }
              frame Default {
                n196 = property on="Test Ring" class="Ring (strict)"("Visible"=FALSE) -> ()  [unwired: 2 in, 2 out]
                n197 = property on="Test Slider" class="Slide (strict)"("Visible"=FALSE) -> ()  [unwired: 2 in, 2 out]
              }
              frame "Brightness  **", "Color Level  **", "Compression  **", "FPS  **", "Sharpness  **" {
                n198 = call <vilib>:"NT Read Number.vi"("Name"=w332) -> ("Numeric"=w331:dbl)  [unwired: 9 in, 1 out]
                n199 = local write "Test Slider"(w331) -> ()
                n200 = property on="Test Slider" class="Slide (strict)"("Visible"=TRUE, "Scale.Maximum"=100.0 ("Scale.Range:Maximum")) -> ()  [unwired: 2 in, 2 out]
                n201 = property on="Test Ring" class="Ring (strict)"("Visible"=FALSE) -> ()  [unwired: 2 in, 2 out]
              }
            }
          }
        }
        n202 = property on="Progress" class="Clust (strict)"("Visible"=FALSE) -> ()  [unwired: 2 in, 2 out]
      }
      event "Test Name": Mouse Enter {
        # "Populate the ring with the list of tests"
        n203 = event-data() -> ()  [unwired: 1 in, 1 out]
        n204 = call <vilib>:"NT Read String Array.vi"("Name"="/TestMode/TestList") -> ("String Array"=w341:string[])  [unwired: 9 in, 1 out]
        n205 = Build Array (concatenate)("Select the test to run...", w341) -> (w340:string[])
        n206 = property on="Test Name" class="Ring (strict)"("Strings []"=w340) -> ()  [unwired: 2 in, 2 out]
      }
      event "Test Name": Value Change {
        w344 = FALSE ("Visible")
        # "Tell the robot the test name to run"
        n207 = event-data() -> ("NewVal"=w348:u16)  [unwired: 1 in]
        n208 = property on="Test Name" class="Ring (strict)"() -> ("Strings []"=w349:string[])  [unwired: 2 in, 2 out]
        n209 = local write "Progress"(T7 {"Test Progress"=0, "Test Progress Text"=""} ("Progress")) -> ()
        n210 = Index Array(array=w349, index=w348) -> (element=w347:string)
        n211 = call <vilib>:"NT Write String.vi"("String"=w347, "Name"="/TestMode/TestName") -> ()  [unwired: 9 in, 1 out]
        n212 = property on="Progress" class="Clust (strict)"("Visible"=TRUE) -> ()  [unwired: 2 in, 2 out]
        n213 = property on="Motor" class="Clust (strict)"("Visible"=w344) -> ()  [unwired: 2 in, 2 out]
        n214 = property on="Test Slider" class="Slide (strict)"("Visible"=w344) -> ()  [unwired: 2 in, 2 out]
        n215 = property on="On/Off" class="Bool (strict)"("Visible"=w344) -> ()  [unwired: 2 in, 2 out]
        n216 = property on="Rev/Fwd" class="Clust (strict)"("Visible"=w344) -> ()  [unwired: 2 in, 2 out]
        n217 = property on="Test Ring" class="Ring (strict)"("Visible"=w344) -> ()  [unwired: 2 in, 2 out]
      }
      event "Select Auto": Mouse Enter {
        # "Populate the combo box with the list of autonomous options"
        n218 = event-data() -> ()  [unwired: 1 in, 1 out]
        n219 = call <vilib>:"NT Read String Array.vi"("Name"="Auto List") -> ("String Array"=w351:string[])  [unwired: 9 in, 1 out]
        n220 = property on="Select Auto" class="CmbBox"("Strings[]"=w351) -> ()  [unwired: 2 in, 2 out]
      }
      event "Select Auto": Value Change {
        # "User modified the Auto Selection. Write to NT variable so robot knows."
        n221 = event-data() -> ("NewVal"=w355:string)  [unwired: 1 in]
        n222 = call <vilib>:"NT Write String.vi"("String"=w355, "Name"="Auto Selector") -> ()  [unwired: 9 in, 1 out]
      }
      event "Command Selection": Value Change {
        # "Get the params and show in table"
        n223 = event-data() -> ("NewVal"=w362:i32)  [unwired: 1 in]
        n224 = property on="Command Selection" class="MCListbox (strict)"() -> ("ItemNames"=w360:string[][])  [unwired: 2 in, 2 out]
        n225 = call <vilib>:"WPI_DashboardUpdate Command Params.vi"("NewVal"=w362, "Commands"=w360, "Param Tbl"=w361) -> ()  [unwired: 8 in, 1 out]
      }
      event "Execute Command": Value Change {
        # "Started one, Unique ID holds\nresponse"
        n226 = event-data() -> ()  [unwired: 1 in, 1 out]
        n227 = property on="Command Selection" class="MCListbox (strict)"() -> ("ItemNames"=w374:string[][])  [unwired: 2 in, 2 out]
        n228 = Index Array(array=w374, index (row)="Command Selection", index (col)=0) -> (element=w372:string)
        n229 = call <vilib>:"Invoke Commands.vi"("Command Params"="Command Params", "Function Name"=w372) -> ("Params"=w368:u8, "Started"=w367:bool)  [unwired: 7 in, 1 out]
        n230 = Array Subset(array="Command Params", length (row)=w368) -> (w369:string[][])  [unwired: 3 in]
        n231 = Select(t="Executing" ("Cmd Status"), s=w367, f="" ("Cmd Status")) -> (s? t:f=→"Cmd Status":string)
      }
      event "Command Selection": Double Click {
        n232 = event-data() -> ("Row"=w384:i32)  [unwired: 1 in]
        n233 = property on="Command Selection" class="MCListbox (strict)"() -> ("ItemNames"=w387:string[][])  [unwired: 2 in, 2 out]
        n234 = local read "Command Params"() -> (w382:string[][])
        n235 = Index Array(array=w387, index (row)=w384, index (col)=0) -> (element=w385:string)
        n236 = call <vilib>:"Invoke Commands.vi"("Command Params"=w382, "Function Name"=w385) -> ("Params"=w381:u8, "Started"=w376:bool)  [unwired: 7 in, 1 out]
        n237 = Array Subset(array=w382, length (row)=w381) -> (w380:string[][])  [unwired: 3 in]
        n238 = Select(t="Executing" ("Cmd Status"), s=w376, f="" ("Cmd Status")) -> (s? t:f=w377:string)
        n239 = local write "Cmd Status"(w377) -> ()
      }
      event "CheckList": Double Click {
        # "Shift clears all"
        # "Update symbols on the listbox"
        n240 = event-data() -> ("PlatMods.Shift"=w390:bool, "Row"=w392:i32)  [unwired: 1 in]
        n241 = case shown="True" w390 {
          tunnel: w392 -> [w396 _]
          tunnel: 1 -> [w395 _]
          frame False {
            n242 = property on="CheckList" class="LstBox (strict)"() -> ("Item Symbols"=w394:i32[])  [unwired: 2 in, 2 out]
            n243 = Replace Array Subset(array=w394, new element=w395, index=w396) -> (w393:i32[])
            n244 = property on="CheckList" class="LstBox (strict)"("Item Symbols"=w393) -> ()  [unwired: 2 in, 2 out]
          }
          frame True {
            w397 = 0 ("Top Row")
            n245 = property on="CheckList" class="LstBox (strict)"() -> ("Number of Rows"=w399:u32)  [unwired: 2 in, 2 out]
            n246 = Initialize Array(0, w399) -> (w398:i32[])
            n247 = property on="CheckList" class="LstBox (strict)"("Top Row"=w397, "Value"=w397, "Item Symbols"=w398) -> ()  [unwired: 2 in, 2 out]
          }
        }
      }
      event "CheckList": Key Down {
        # "Update symbols on the listbox\nLeft and right keys check and uncheck"
        n248 = event-data() -> ("VKey"=w404:T22)  [unwired: 1 in]
        n249 = case shown="\"Left\", \"Right\"" w404 {
          selector: w404 -> [w409 _]
          tunnel: eventvkey."Left" ("VKey") -> [w407 _]
          frame "Left", "Right" {
            n250 = Equal?(x=w407, y=w409) -> (x = y?=w408:bool)
            n251 = Select(t=0, s=w408, f=1) -> (s? t:f=w410:i32)
            n252 = property on="CheckList" class="LstBox (strict)"() -> ("Item Symbols"=w413:i32[])  [unwired: 2 in, 2 out]
            n253 = Replace Array Subset(array=w413, new element=w410, index="CheckList") -> (w412:i32[])
            n254 = property on="CheckList" class="LstBox (strict)"("Item Symbols"=w412) -> ()  [unwired: 2 in, 2 out]
          }
          frame Default {
          }
        }
      }
      event "DB Camera Config": Value Change {
        # "Show or hide the cluster of controls, store in ini file"
        n255 = event-data() -> ("NewVal"=w418:bool)  [unwired: 1 in]
        n256 = case shown="False" w418 {
          tunnel: w417 -> [w427 _]
          tunnel: [w420 w438] -> w416
          tunnel: w415 -> [w419 w438]
          frame False {
            w434 = "Camera"
            w437 = FALSE ("Visible")
            n257 = local read "Camera Settings"() -> (w426:T2)
            n258 = Index Array(array=w427) -> (element=w430:cluster{string[]})  [unwired: 1 in]
            n259 = Unbundle(w426) -> ("Frame Rate"=w425:i32, "Compression"=w424:i32, "Size"=w428:u16)
            n260 = Unbundle(w430) -> (w429:string[])
            n261 = Index Array(array=w429, index=w428) -> (element=w423:string)
            n262 = call-poly <vilib>:"Write Key.vi"("section"=w434, "value"=w423, "key"="Size", "refnum"=w419) -> ("refnum out"=w436:T20)  [unwired: 2 in, 5 out]
            n263 = call-poly <vilib>:"Write Key.vi"("section"=w434, "value"=w425, "key"="FrameRate", "refnum"=w436) -> ("refnum out"=w435:T20)  [unwired: 1 in, 6 out]
            n264 = property on="Camera Settings" class="Clust (strict)"("Visible"=w437) -> ()  [unwired: 2 in, 2 out]
            n265 = local write "DB Camera Config"(w437) -> ()
            n266 = call-poly <vilib>:"Write Key.vi"("section"=w434, "value"=w424, "key"="Compression", "refnum"=w435) -> ("refnum out"=w421:T20)  [unwired: 1 in, 6 out]
            n267 = call <vilib>:"Close Config Data.vi"("refnum"=w421) -> ("file path"=w422:path)  [unwired: 2 in, 8 out]
            n268 = call <vilib>:"Open Config Data.vi"("configuration file path"=w422) -> ("refnum"=w420:T20)  [unwired: 8 in, 2 out]
          }
          frame True {
            n269 = property on="Camera Settings" class="Clust (strict)"("Visible"=TRUE) -> ()  [unwired: 2 in, 2 out]
          }
        }
      }
      event "Camera Settings": Value Change {
        # "Update summary string when any elements of DB camera change"
        n270 = event-data() -> ("NewVal"=w452:T2)  [unwired: 1 in]
        n271 = Index Array(array=w448) -> (element=w447:cluster{string[]})  [unwired: 1 in]
        n272 = Unbundle(w452) -> ("Frame Rate"=w443:i32, "Compression"=w442:i32, "Size"=w445:u16)
        n273 = Unbundle(w447) -> (w446:string[])
        n274 = Index Array(array=w446, index=w445) -> (element=w444:string)
        n275 = Format Into String(format string="%s   %dfps   %d%%", w444, w443, w442) -> (resulting string=w449:string)  [unwired: 2 in, 1 out]
        n276 = Build Array(w449) -> (w450:string[])
        n277 = property on="DB Camera Config" class="Bool (strict)"("Strings [4]"=w450) -> ()  [unwired: 2 in, 2 out]
      }
      event "Motor.Enable": Value Change {
        # "When the test mode otor enable helper is set, update that\ntree row item's value"
        n278 = event-data() -> ("NewVal"=w459:bool)  [unwired: 1 in]
        n279 = Unbundle("Motor") -> ("Value"=w458:dbl)  [unwired: 1 out]
        n280 = Select(t=w458, s=w459, f=0.0) -> (s? t:f=w456:dbl)
        n281 = call <vilib>:"NT Write Number.vi"("Numeric"=w456, "Name"=w455) -> ()  [unwired: 9 in, 1 out]
      }
      event "Test Slider": Value Change {
        # "When the test mode slider helper is set, update that\ntree row item's value"
        n282 = event-data() -> ("NewVal"=w463:dbl)  [unwired: 1 in]
        n283 = call <vilib>:"NT Write Number.vi"("Numeric"=w463, "Name"=w464) -> ()  [unwired: 9 in, 1 out]
      }
      event "On/Off": Value Change {
        # "When the test mode on/off helper value is set, update that\ntree row item's value"
        n284 = event-data() -> ("NewVal"=w469:bool)  [unwired: 1 in]
        n285 = Boolean To (0,1)(Boolean=w469) -> (0, 1=w468:i16)
        n286 = call <vilib>:"NT Write Number.vi"("Numeric"=w468, "Name"=w467) -> ()  [unwired: 9 in, 1 out]
      }
      event "Rev/Fwd": Value Change {
        # "When the test mode helper value for relays is set, update that\ntree row item's value"
        n287 = event-data() -> ("NewVal.Forward"=w478:bool, "NewVal.Reverse"=w477:bool)  [unwired: 1 in]
        n288 = Boolean To (0,1)(Boolean=w478) -> (0, 1=w474:i16)
        n289 = Boolean To (0,1)(Boolean=w477) -> (0, 1=w476:i16)
        n290 = Negate(x=w476) -> (-x=w475:i16)
        n291 = Add(x=w474, y=w475) -> (x+y=w473:i16)
        n292 = call <vilib>:"NT Write Number.vi"("Numeric"=w473, "Name"=w472) -> ()  [unwired: 9 in, 1 out]
      }
      event "Test Ring": Value Change {
        # "When a test mode helper value is selected from the ring,\nset the tree item's variable to the string value"
        n293 = event-data() -> ("NewVal"=w483:u16)  [unwired: 1 in]
        n294 = property on="Test Ring" class="Ring (strict)"() -> ("Strings []"=w484:string[])  [unwired: 2 in, 2 out]
        n295 = Index Array(array=w484, index=w483) -> (element=w482:string)
        n296 = call <vilib>:"NT Write String.vi"("String"=w482, "Name"=w481) -> ()  [unwired: 9 in, 1 out]
      }
      event "Rec Mode": Value Change {
        # "Update globals for recording mode and path to read log from.\nClear when logging and let NetworkTables set path for vision to\nuse."
        n297 = event-data() -> ("NewVal"=w496:enum32{"Stop", "Record", "Playback"})  [unwired: 1 in]
        n298 = global write "WPI_DashboardLogging Global.vi" "Logging Filename"(path "") -> ()
        n299 = global write "WPI_DashboardLogging Global.vi" "Recording"(w496) -> ()
        n300 = case shown="\"Playback\"" w496 {
          tunnel: w495 -> [_ w498 w507]
          tunnel: [_ _ w506] -> w492
          tunnel: [_ _ w505] -> _
          tunnel: w490 -> [_ _ w503]
          tunnel: cluster{i32, i32} {-250, 170} -> [_ _ w502]
          tunnel: [_ _ T23 {"Image Size"=TRUE, "Image Type"=TRUE, "Pixel Value"=TRUE, "ROI Information"=TRUE, "Zoom Factor"=FALSE} ("Image Information Shown:All Elements")] -> w488
          tunnel: [_ _ TRUE ("Zoom Factor")] -> w487
          tunnel: w486 -> [_ _ w499]
          frame Default {
          }
          frame "Stop", "Record" {
            # "Place Window too"
            n301 = invoke class="VI" method="FP.Close"(reference=w498) -> (reference out=w497:refnum<vi>)  [unwired: 2 in, 2 out]
            n302 = invoke class="VI" method="Abort VI"(reference=w497) -> ()  [unwired: 2 in, 3 out]
          }
          frame "Playback" {
            n303 = call "Open Playback Panel.vi"("Offset"=w502, "DB VI Ref"=w503, "Playback in"=w507) -> ("Playback out"=w504:refnum<vi>)  [unwired: 8 in]
            n304 = register-events(w504, w499) -> (reference out=w506:refnum<event-registration>, error out=w505:errorcluster)  [unwired: 2 in]
          }
        }
        n305 = property on="Camera Image" class="ImageControl"("Image Information Shown"=w488, "Image Information Visible"=w487) -> ()  [unwired: 2 in, 2 out]
        n306 = call <vilib>:"WPI_DashboardNT Log FieldName Cache.vi"("Operation"=enum16{"Lookup/Add", "Index", "Clear"}."Clear") -> ()  [unwired: 8 in, 3 out]
      }
      event Panel Close {
        w509 = enum32{"Stop", "Record", "Playback"}."Stop" ("Rec Mode")
        # "Playback window has been closed, abort"
        n307 = event-data() -> ()  [unwired: 1 in, 4 out]
        n308 = local write "Rec Mode"(w509) -> ()
        n309 = global write "WPI_DashboardLogging Global.vi" "Recording"(w509) -> ()
      }
      event Panel Close {
        # "Abort playback window and ourself"
        n310 = event-data() -> ()  [unwired: 1 in, 4 out]
        n311 = invoke class="VI" method="FP.Close"(reference=w515) -> (reference out=w514:refnum<vi>)  [unwired: 2 in, 2 out]
        n312 = invoke class="VI" method="Abort VI"(reference=w514) -> (error out=w513:errorcluster)  [unwired: 2 in, 2 out]
        n313 = invoke class="VI" method="Abort VI"(error in=w513) -> ()  [unwired: 2 in, 3 out]
      }
      event User Event {
        n314 = event-data() -> ("IDs"=w523:cluster{"RPC field ID":u16, "Unique ID":u16}, "String"=w522:string)  [unwired: 1 in]
        n315 = Bundle("IDs"=w523, "String"=w522) -> (w521:T9)  [unwired: 1 in]
        n316 = call <vilib>:"Retrieve RPC Response.vi"("RPC Response"=w521) -> ("Output"=w518:string[][])  [unwired: 10 in]
        n317 = Build Array (concatenate)(w516, w518) -> (w517:string[][])
        n318 = local write "Command Params"(w517) -> ()
        n319 = local write "Cmd Status"("" ("Cmd Status")) -> ()
      }
      event "Vision": Value Change {
        # "Enable/Disable Compression slider.\nHW USB is hard-coded into the camera"
        n320 = event-data() -> ("NewVal"=w530:u16)  [unwired: 1 in]
        n321 = Equal?(x=w530, y=u32 2 ("milliseconds to wait")) -> (x = y?=w528:bool)
        n322 = Select(t=T24."Disabled and Grayed Out" ("Disabled"), s=w528, f=T24."Enabled" ("Disabled")) -> (s? t:f=w525:T24)
        n323 = property on="Compression" class="Slide (strict)"("DisabledEnum"=w525) -> ()  [unwired: 2 in, 2 out]
      }
      event "Tree": Double Click {
        n324 = event-data() -> ("PlatMods"=w535:T27, "Tag"=w534:string)  [unwired: 1 in]
        n325 = Unbundle(w535) -> ("Shift"=w533:bool)  [unwired: 4 out]
        n326 = Not(x=w533) -> (.not. x?=w532:bool)
        n327 = call <vilib>:"NT Update Persistence.vi"("Persistence"=w532, "Name"=w534) -> ()  [unwired: 9 in, 1 out]
      }
    }
  }
  n328 = while {
    tunnel: w47 -> [w539]
    i -> [w542]
    stop <- FALSE stop-if-true
    n329 = Wait (ms)(milliseconds to wait=u32 100) -> ()  [unwired: 1 out]
    n330 = case shown="\"Playback\"" "Rec Mode" {
      tunnel: w542 -> [_ _ w557]
      tunnel: [u32 2829099 ("Base Color") u32 11141120 ("Target Color") w546] -> w538
      frame "Stop", Default {
        # "Reset the color, extra updates don't cost much"
      }
      frame "Record" {
      }
      frame "Playback" {
        # "Playback"
        n331 = Quotient & Remainder(x=w557, y=u32 50 ("milliseconds to wait")) -> (x-y*floor(x/y)=w553:u32)  [unwired: 1 out]
        n332 = Divide(x=w553, y=u32 50 ("milliseconds to wait")) -> (x/y=w550:dbl)
        n333 = Multiply(x=6.283185307179586, y=w550) -> (x*y=w555:dbl)
        n334 = Sine(x=w555) -> (sin(x)=w554:dbl)
        n335 = Absolute Value(x=w554) -> (abs(x)=w547:dbl)
        n336 = call "Interpolate RGB Color.vi"("Proportion"=w547, "Target Color"=u32 30976, "Base Color"=u32 2829099) -> ("Result Color"=w546:u32)  [unwired: 8 in]
      }
    }
    n337 = property class="Pane"(reference=w539, "PaneColor"=w538) -> ()  [unwired: 1 in, 2 out]
  }
  n338 = local write "Dashboard Tab"(T1."Drive" ("Dashboard Tab")) -> ()
  n339 = property on="On/Off" class="Bool (strict)"("Visible"=w15) -> ()  [unwired: 2 in, 2 out]
  n340 = property on="Motor" class="Clust (strict)"("Visible"=w15) -> ()  [unwired: 2 in, 2 out]
  n341 = property on="Progress" class="Clust (strict)"("Visible"=w15) -> ()  [unwired: 2 in, 2 out]
  n342 = property on="Test Ring" class="Ring (strict)"("Visible"=w15) -> ()  [unwired: 2 in, 2 out]
  n343 = property on="Rev/Fwd" class="Clust (strict)"("Visible"=w15) -> ()  [unwired: 2 in, 2 out]
  n344 = property on="Camera Settings" class="Clust (strict)"("Visible"=w15) -> ()  [unwired: 2 in, 2 out]
  n345 = while {
    tunnel: u16 1741 ("timeout ms (25000)") -> [w559]
    stop <- FALSE stop-if-true
    n346 = TCP Create Listener(10:w559) -> (0:w558:errorcluster, 3:w560:refnum<k5>)  [unwired: 4 in, 1 out]
    n347 = case shown="No Error" w558 {
      selector: w558 -> [w562 _]
      tunnel: w560 -> [w563 _]
      frame No Error {
        n348 = while {
          tunnel: w563 -> [w566]
          tunnel: w562 -> [w565]
          stop <- FALSE stop-if-true
          n349 = TCP Wait On Listener(8:w565, 11:w566) -> (0:w567:errorcluster, 4:w568:refnum<k5>)  [unwired: 2 in, 3 out]
          n350 = local write "TCP"(w568) -> ()
          n351 = case shown="No Error" w567 {
            frame No Error {
            }
            frame Error {
              n352 = Wait (ms)(milliseconds to wait=u32 1000) -> ()  [unwired: 1 out]
            }
          }
        }
      }
      frame Error {
        n353 = Wait (ms)(milliseconds to wait=u32 1000) -> ()  [unwired: 1 out]
      }
    }
  }
  n354 = local write "DB Camera Config"(w15) -> ()
  n355 = local write "Command Params"(string[][] [] ("Command Params")) -> ()
  n356 = global write "WPI_DashboardLogging Global.vi" "Recording"(w41) -> ()
  n357 = local write "Command Selection"(u16 0 ("milliseconds to wait")) -> ()
  n358 = local write "Rec Mode"(w41) -> ()
